vi "Master Setup Read Write Setup Paths.vi"(8 "error in (no error)":errorcluster, 9 "Read (F)/Write (T)":bool, 10 "Pattern Label":T1 items=["Channel Setup (0)", "PID Setup (1)", "Filter Setup (2)", "~Reserved Old CAN Msgs (3)", "~Reserved Old CAN1 (4)", "~Reserved Old CAN2 (5)", "Digital Inputs Setup (6)", "Digital Outputs Setup (7)", "Logging 1 Setup (8)", "Logging 2 Setup (9)", "Logging 3 Setup (10)", "Setpoint Setup (11)", "Test Series Setup (12)", "Graph Setup (13)", "System Configure (14)", "Header (15)", "Profile Manager (16)", "Post-Mortem Logging (17)", "High-Speed Data (18)", "Statistic Channel Setup (19)", "Ramp Channel Setup (20)", "ETAS INCA Channel Setup (21)", "ETC ECCS Transducer Setup (22)", "ETC ECCS Test Setup (23)", "AVL AK Smoke Meter Setup (24)", "Triggers Setup (25)", "Alarm Limits Setup (26)", "YKWT1 Measurement (27)", "YKWT1 Instrument (28)", "Auto File Settings (29)", "Playback File Setting (30)", "UUT Constants (31)", "UPS Setup (32)", "Differential Channel Setup (33)", "Integral Channel Setup (34)", "Signal Channel Setup (35)", "Calibration Setup (36)", "BNC Setup (37)", "ASAP3 Setup (38)", "Chassis Force Calculations (39)", "Chassis Teststand Losses (40)", "Chassis Vehicle Losses (41)", "Formula Channels (42)", "ASAP3 Map Coords Setup (43)", "Digital Controls Setup (44)", "Push Buttons Setup (45)", "Sliders Setup (46)", "~Reserved~ (47)", "Email Setup (48)", "Timer Setup (49)", "Unit Conversion Setup (50)", "Visible Channels (51)", "Main Display Setup (52)", "Message Display Setup (53)", "Input Display Setup (54)", "Unico Parameter Downloads (55)", "Flow Meter Setup (56)", "Channel Zero Offset (57)", "YKWT2 Measurement (58)", "YKWT2 Instrument (59)", "~Reserved Old CAN3 (60)", "CAS Setup (61)", "Accumulation Channel Setup (62)", "Valvetrain Dynamics Setup (63)", "CCP Setup (64)", "System Log Setup (65)", "Throttle Controller (66)", "RE Shifter (67)", "Main Display (68)", "~Reserved~ (69)", "FlexRay (70)", "YKWT3 Measurement (71)", "YKWT3 Instrument (72)", "CAN XNET API (73)"], 11 "Master Setup File Path (in)":path) -> (0 "error out":errorcluster, 1 "Old Setup Paths":path[](array[path]), 2 "New Setup Paths":path[](array[path]), 3 "New Setup Path":path, 4 "Old Setup Path":path)   [LabVIEW 2017]
uses:
  Master Setup Pattern Enum.ctl
panel:
  in  "Setup File (System Configure)":path=path "C:/Revolutionary Engineering/REPS/Setup Files/Default/GM Trans Cell 2/SystemConfigure GM cell 2.cfs"
  in  "Setup File (Setpoint)":path=path "C:/Revolutionary Engineering/REPS/Setup Files/Default/RE Cell 3-1/re cell 3 setpoints.spt"
  in  "Setup File (CAN 0)":path
  in  "Setup File (CAN 1)":path
  in  "Setup File (Can Message)":path
  in  "Setup File (Playback)":path
  in  "Setup File (UUT Constants)":path
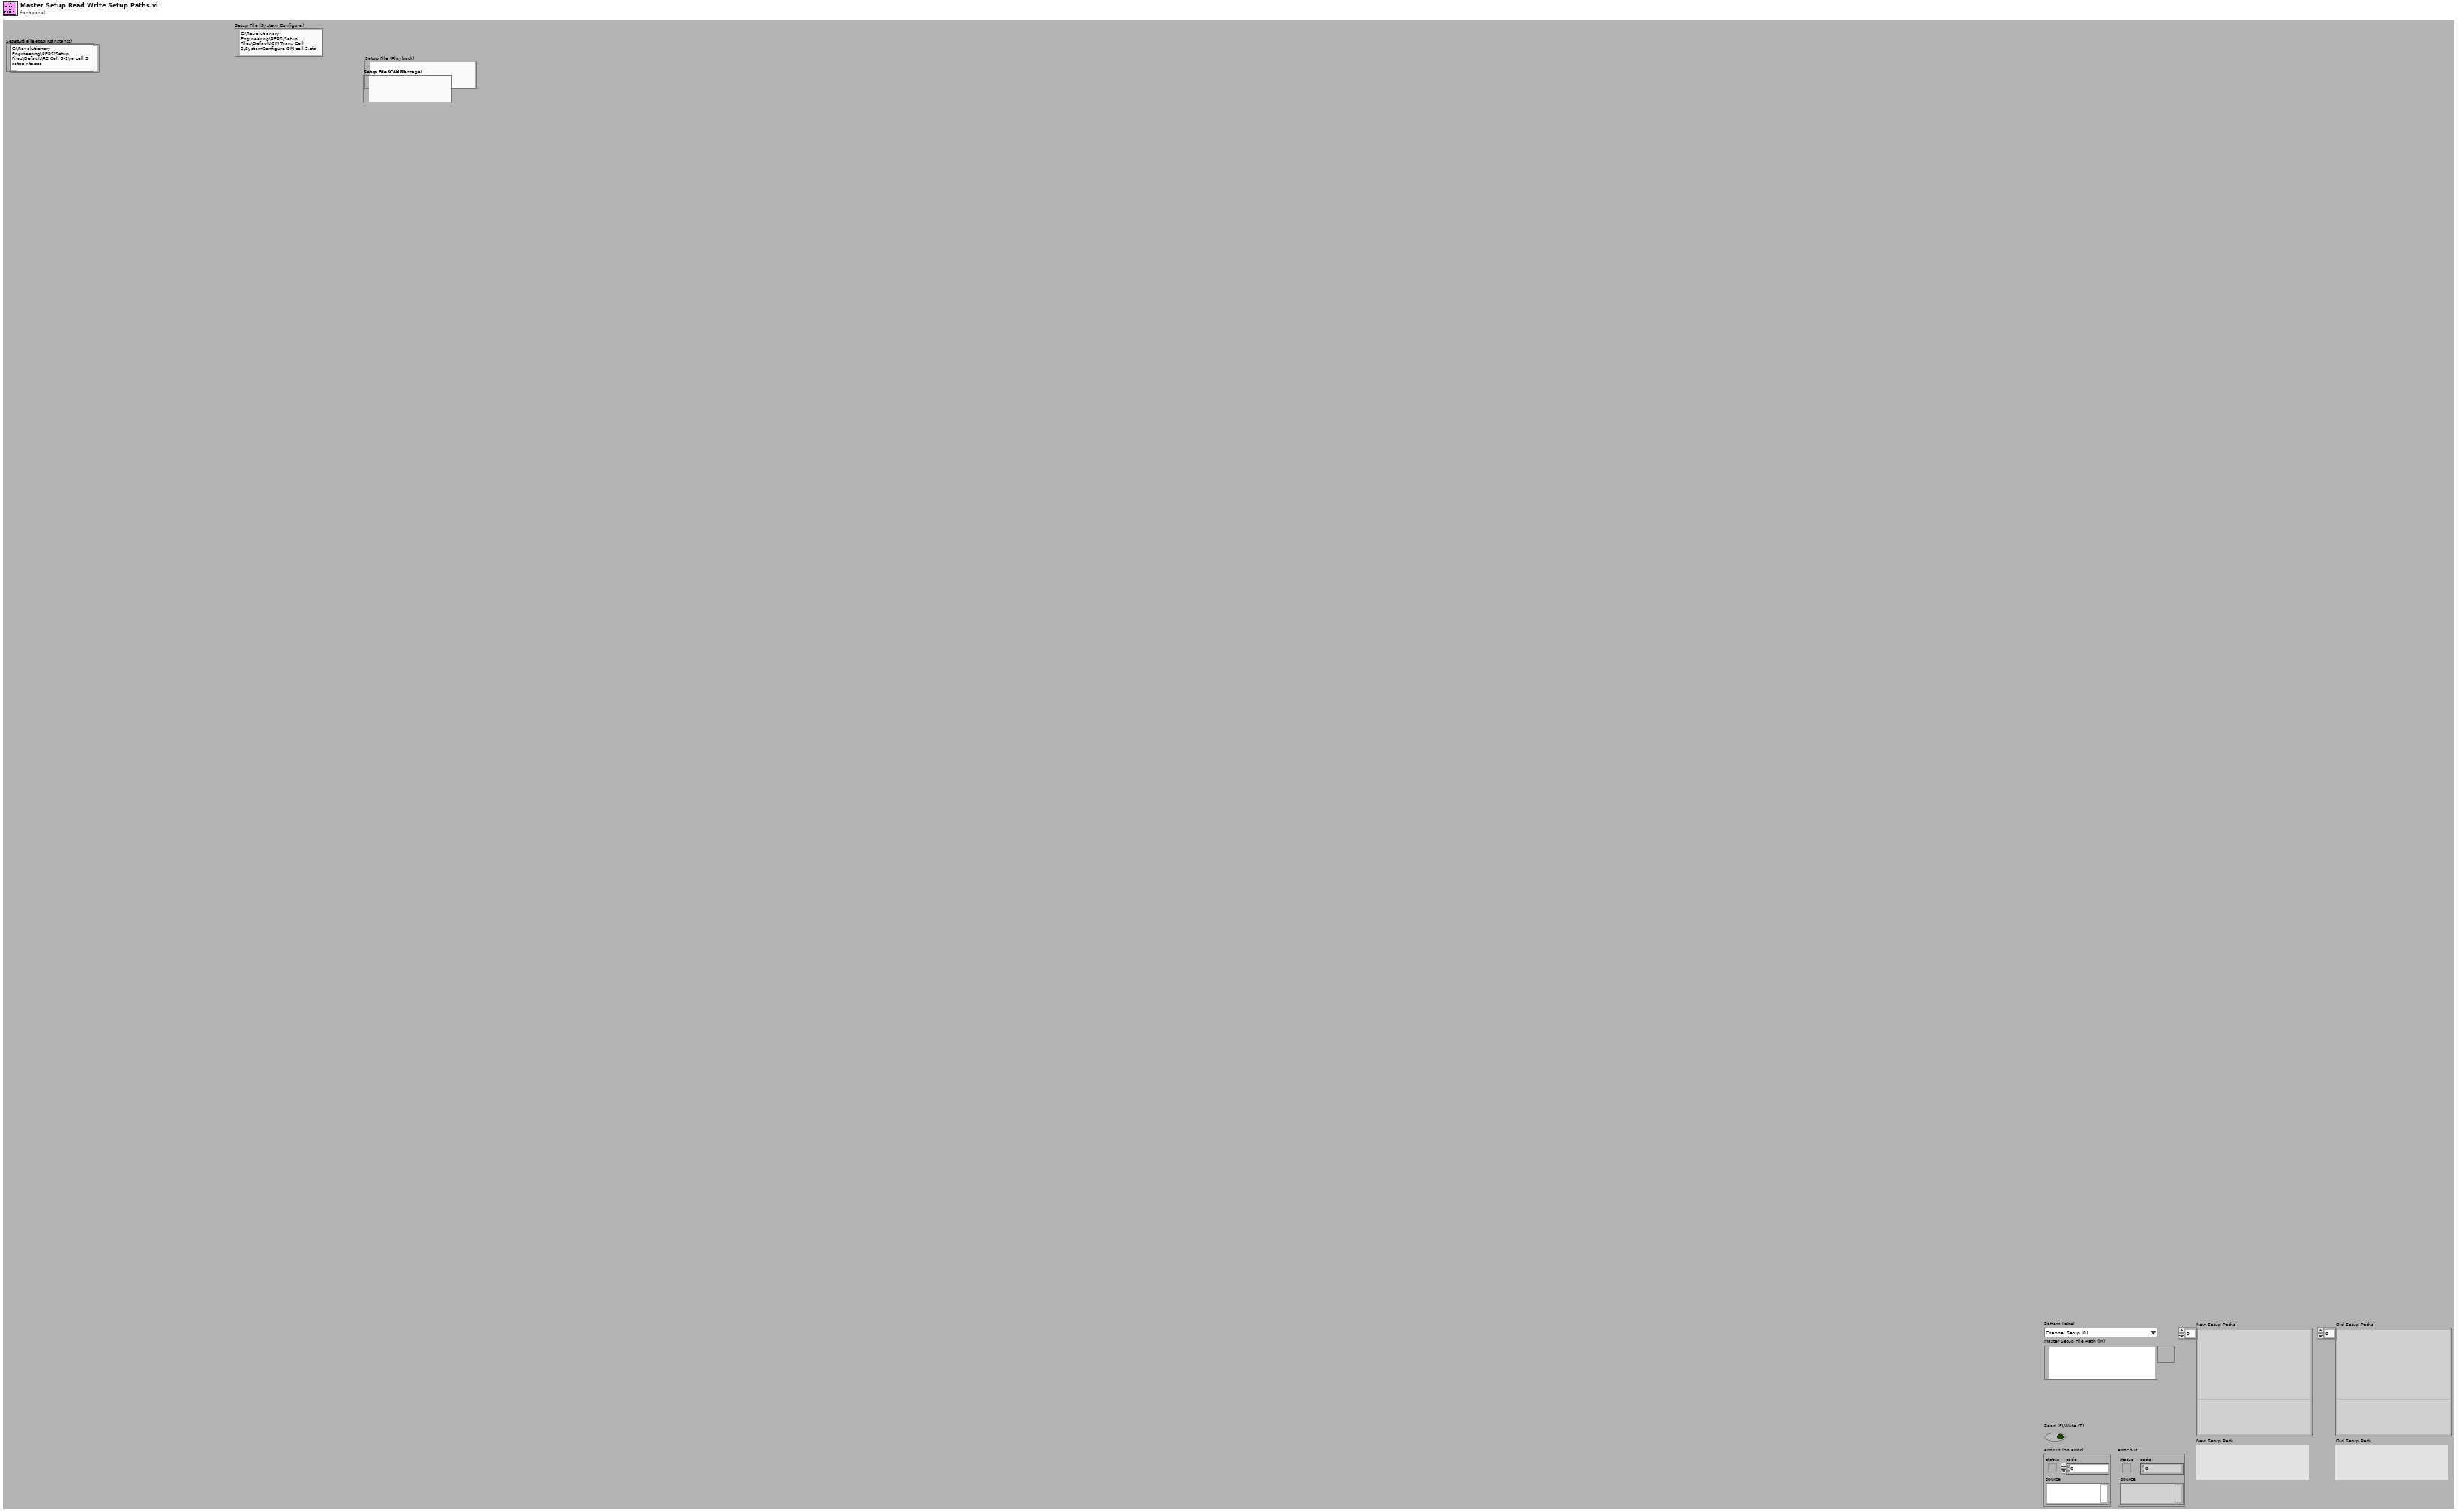
[diagram p1: front panel]
types:
  T1 = typedef "Master Setup Pattern Enum.ctl" = i32
diagram:
  n1 = while {
    shift-right: [w15] -> w2
    shift-left: _ -> [w6]
    shift-right: [w10] -> w1
    shift-left: _ -> [w7]
    stop <- TRUE stop-if-true
    # "Old Setup Paths"
    # "New Setup Paths"
    n2 = Empty Array?(array=w6) -> (empty?=w4:bool)
    n3 = Empty Array?(array=w7) -> (empty?=w8:bool)
    n4 = Or(x=w4, y=w8) -> (x .or. y?=w5:bool)
    n5 = case shown="True" w5 {
      tunnel: w6 -> [w21 _]
      tunnel: [w21 w22] -> w17
      tunnel: w7 -> [w20 _]
      tunnel: [w20 w22] -> w12
      frame False {
      }
      frame True {
        n6 = call "Master Setup Titles.vi"() -> ("Setup Description w/Numbers"=w24:string[])  [unwired: 6 in, 5 out]
        n7 = Array Size(array=w24) -> (size(s)=w23:i32)
        n8 = Initialize Array(path "", w23) -> (w22:path[])
      }
    }
    n9 = To Long Integer(number="Pattern Label") -> (32bit integer=w9:T1)
    n10 = case shown="True" "Read (F)/Write (T)" {
      tunnel: w17 -> [w27 w28]
      tunnel: [w27 w33] -> w15
      tunnel: w9 -> [_ w30]
      tunnel: "Master Setup File Path (in)" -> [_ w34]
      tunnel: w12 -> [w26 w32]
      tunnel: [w26 w31] -> w10
      frame False {
      }
      frame True {
        n11 = Index Array(array=w28, index=w30) -> (element=w29:path)
        n12 = Replace Array Subset(array=w28, new element=w34, index=w30) -> (w33:path[])
        n13 = Replace Array Subset(array=w32, new element=w29, index=w30) -> (w31:path[])
      }
    }
    n14 = Index Array(array=w15, index=w9) -> (element=→"New Setup Path":path)
    n15 = Index Array(array=w10, index=w9) -> (element=→"Old Setup Path":path)
  }
  "New Setup Paths" <- w2
  "Old Setup Paths" <- w1
  "error out" <- "error in (no error)"
